vi "Activate_Panel.vi"(0 "Panel Name":string, 1 "Panel Array":string[](array[string])) -> (2 "Top":i32, 3 "Left":i32, 4 "Active":bool)   [LabVIEW 2018]
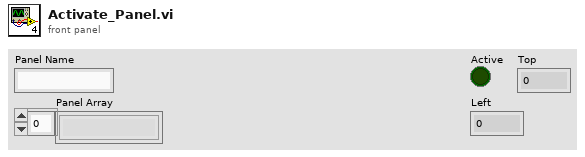
[diagram p1: front panel]
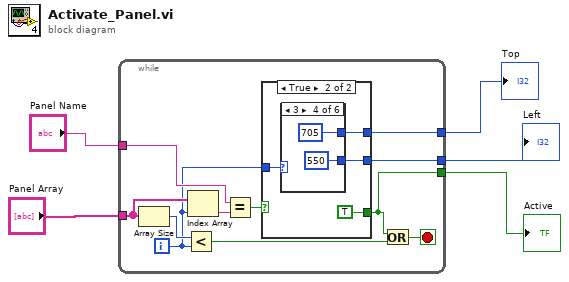
[diagram p0: block diagram]
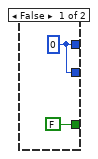
[diagram p2: hidden frame]
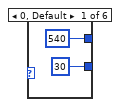
[diagram p3: hidden frame]
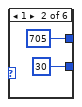
[diagram p4: hidden frame]
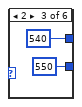
[diagram p5: hidden frame]
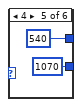
[diagram p6: hidden frame]
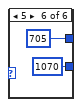
[diagram p7: hidden frame]
diagram:
  n1 = while {
    tunnel: "Panel Name" -> [w15]
    tunnel: "Panel Array" -> [w13]
    tunnel: [w8] -> w3
    tunnel: [w7] -> w2
    tunnel: [w6] -> w1
    i -> [w9]
    stop <- w10 stop-if-true
    n2 = Array Size(array=w13) -> (size(s)=w12:i32)
    n3 = Less?(x=w12, y=w9) -> (x < y?=w11:bool)
    n4 = Index Array(array=w13, index=w9) -> (element=w14:string)
    n5 = Equal?(x=w15, y=w14) -> (x = y?=w16:bool)
    n6 = case shown="True" w16 {
      tunnel: w9 -> [_ w22]
      tunnel: [w18 w21] -> w6
      tunnel: [w18 w20] -> w7
      tunnel: [FALSE TRUE] -> w8
      frame False {
        w18 = 0
      }
      frame True {
        n7 = case shown="3" w22 {
          tunnel: [30 30 550 550 1070 1070] -> w21
          tunnel: [540 705 540 705 540 705] -> w20
          frame 0, Default {
          }
          frame 1 {
          }
          frame 2 {
          }
          frame 3 {
          }
          frame 4 {
          }
          frame 5 {
          }
        }
      }
    }
    n8 = Or(x=w8, y=w11) -> (x .or. y?=w10:bool)
  }
  "Active" <- w3
  "Top" <- w2
  "Left" <- w1
